vi "LunchExperiment.vi"(10 "Run on open":bool, 11 "appended path":path) -> ()   [LabVIEW 2017]
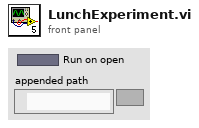
[diagram p1: front panel]
types:
  T1 = enum32{"Invalid", "Standard", "Closed", "Hidden", "Minimized", "Maximized"}
  T2 = enum32{"Bad", "Idle", "Run top level", "Running"}
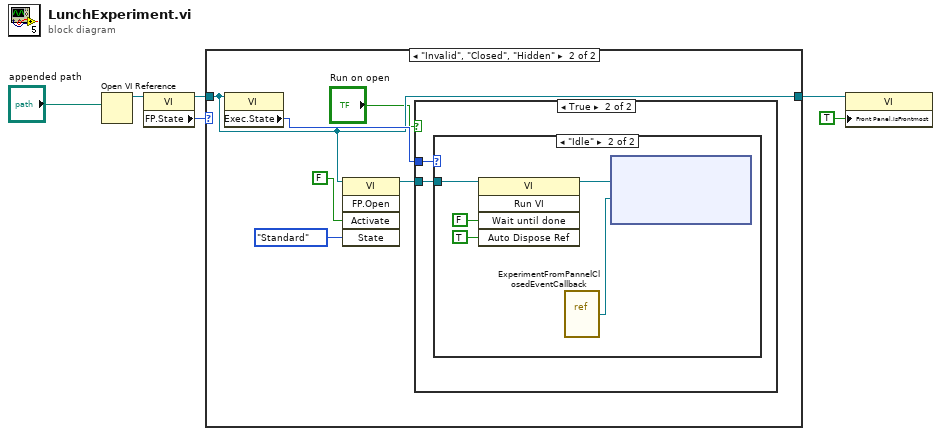
[diagram p0: block diagram]
diagram:
  n1 = Open VI Reference(vi path="appended path") -> (vi reference=w5:refnum<vi>)  [unwired: 5 in, 1 out]
  n2 = property class="VI"(reference=w5) -> (reference out=w1:refnum<vi>, "FP.State"=w4:T1)  [unwired: 1 in, 1 out]
  n3 = case shown="\"Invalid\", \"Closed\", \"Hidden\"" w4 {
    tunnel: [w7 w10] -> w3
    tunnel: w1 -> [w7 w10]
    frame Default {
    }
    frame "Invalid", "Closed", "Hidden" {
      n4 = property class="VI"(reference=w10) -> ("Exec.State"=w12:T2)  [unwired: 1 in, 2 out]
      n5 = invoke class="VI" method="FP.Open"(reference=w10, "Activate"=FALSE ("Activate?"), "State"=T1."Standard") -> (reference out=w9:refnum<vi>)  [unwired: 2 in, 4 out]
      n6 = case shown="True" "Run on open" {
        tunnel: w12 -> [_ w15]
        tunnel: w9 -> [_ w14]
        frame False {
        }
        frame True {
          n7 = case shown="\"Idle\"" w15 {
            tunnel: w14 -> [_ w18]
            frame Default {
            }
            frame "Idle" {
              n8 = invoke class="VI" method="Run VI"(reference=w18, "Wait until done"=FALSE ("Wait Until Done"), "Auto Dispose Ref"=TRUE ("Auto Dispose Reference")) -> (reference out=w16:refnum<vi>)  [unwired: 2 in, 4 out]
              n9 = vi-ref "ExperimentFromPannelClosedEventCallback.vi"() -> ("vi reference"=w17:refnum<vi>)
              n10 = node(w16, w17) -> ()  [unwired: 3 in, 2 out]
            }
          }
        }
      }
    }
  }
  n11 = property class="VI"(reference=w3, "Front Panel.IsFrontmost"=TRUE ("Front Panel Window:Is Frontmost")) -> ()  [unwired: 1 in, 2 out]
